vi "get_LBO_status.vi"(8 "error in (no error)":errorcluster, 11 "VISA resource name":refnum<visa-resource-name>) -> (0 "error out":errorcluster, 2 "LBO status":bool, 3 "VISA resource name out":refnum<visa-resource-name>)   [LabVIEW 2013]
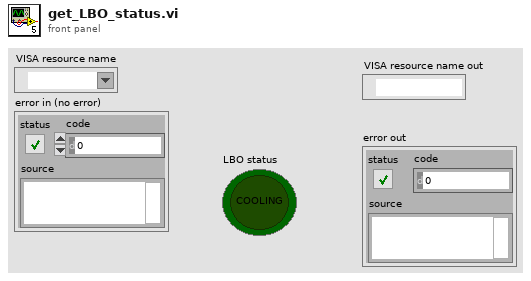
[diagram p1: front panel]
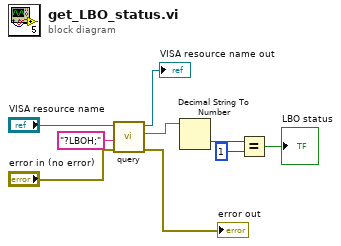
[diagram p0: block diagram]
diagram:
  n1 = call "query.vi"("error in (no error)"="error in (no error)", "write buffer"="?LBOH;", "VISA resource name"="VISA resource name") -> ("error out"=→"error out":errorcluster, "substring"=w4:string, "VISA resource name out"=→"VISA resource name out":refnum<visa-resource-name>)  [unwired: 6 in]
  n2 = Decimal String To Number(string=w4) -> (number=w3:i32)  [unwired: 2 in, 1 out]
  n3 = Equal?(x=w3, y=1) -> (x = y?=→"LBO status":bool)
